vi "load images.vi"(0 "selected data path":path, 1 "DataMarijnFormat":bool=TRUE, 7 "Data(T)orLUT(F)?":bool, 11 "error in":errorcluster, 12 "frame no.":i32) -> (3 "image name":string, 4 "String":string, 6 "Image Out":T1, 10 "framenumber":i32, 14 "error out":errorcluster, 15 "frametime":i32)   [LabVIEW 2011, in "OfflineTracker.lvlib"]
uses:
  <vilib>/vision/Image Controls.llb/IMAQ Image.ctl
  <vilib>/Utility/file.llb/Read From Spreadsheet File (string).vi
  <vilib>/Utility/file.llb/Read From Spreadsheet File (DBL).vi
  OfflineTracker.lvlib
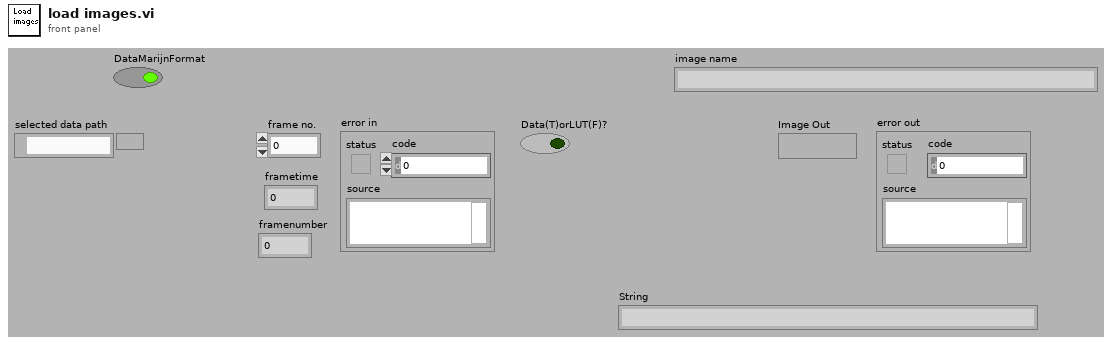
[diagram p1: front panel]
types:
  T1 = typedef "IMAQ Image.ctl" = refnum<image>
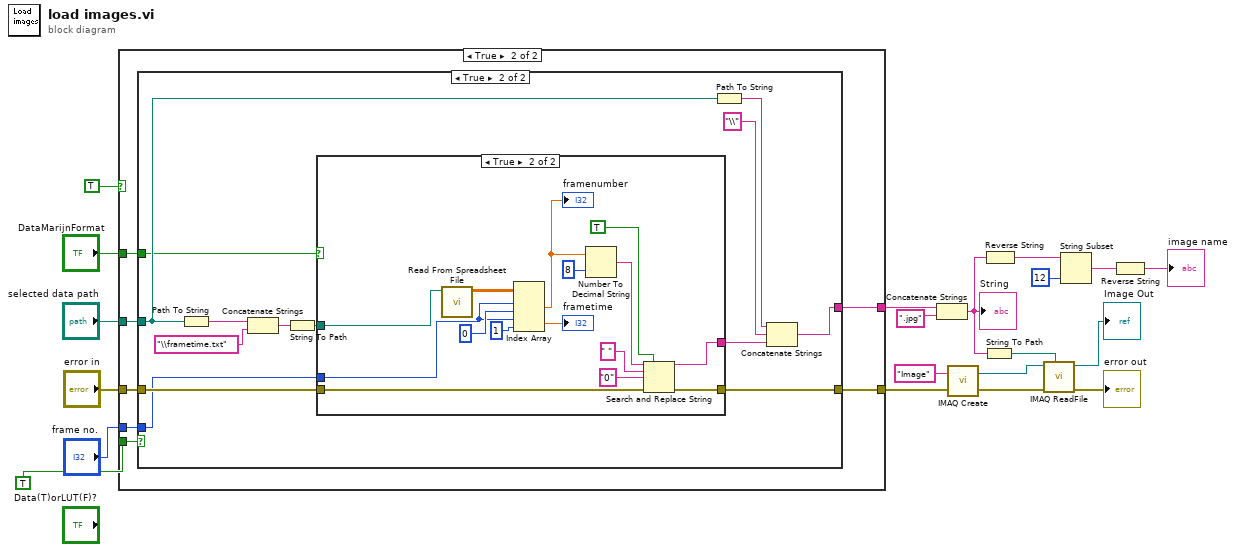
[diagram p0: block diagram]
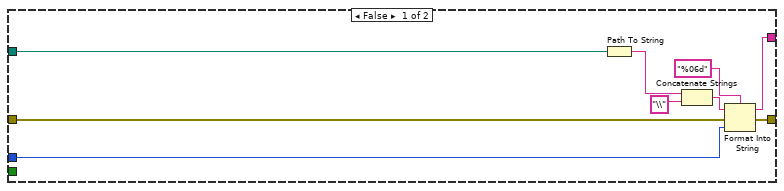
[diagram p2: hidden frame]
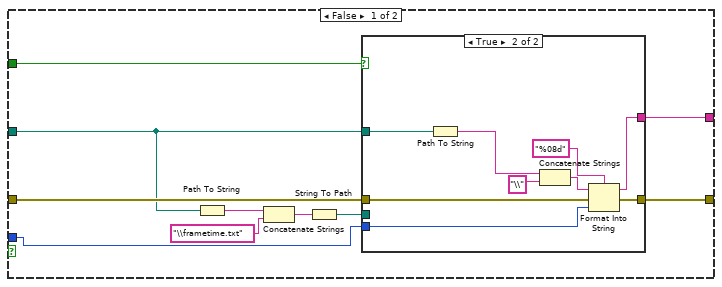
[diagram p3: hidden frame]
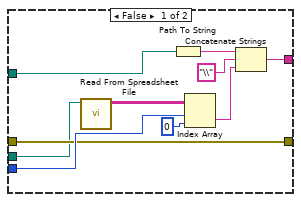
[diagram p4: hidden frame]
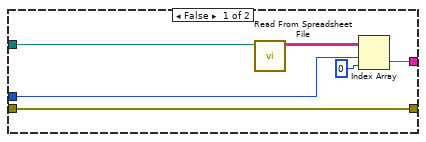
[diagram p5: hidden frame]
diagram:
  n1 = case shown="True" TRUE {
    tunnel: "selected data path" -> [w27 w36]
    tunnel: "error in" -> [w29 w34]
    tunnel: [w28 w33] -> w17
    tunnel: [w26 w35] -> w16
    tunnel: "frame no." -> [w25 w32]
    tunnel: TRUE ("Data(T)orLUT(F)?") -> [_ w31]
    tunnel: "DataMarijnFormat" -> [_ w30]
    frame False {
      n2 = Path To String(path=w27) -> (string=w21:string)
      n3 = Concatenate Strings(w21, "\\" ("string")) -> (w22:string)
      n4 = Format Into String(format string="%06d", initial string=w22, error in=w29, w25) -> (resulting string=w26:string, error out=w28:errorcluster)
    }
    frame True {
      n5 = case shown="True" w31 {
        tunnel: w36 -> [w38 w68]
        tunnel: [w43 w77] -> w35
        tunnel: w34 -> [w46 w74]
        tunnel: [w45 w73] -> w33
        tunnel: w32 -> [w44 w67]
        tunnel: w30 -> [w42 w66]
        frame False {
          n6 = Path To String(path=w38) -> (string=w41:string)
          n7 = Concatenate Strings(w41, "\\frametime.txt" ("string")) -> (w40:string)
          n8 = String To Path(string=w40) -> (path=w37:path)
          n9 = case shown="True" w42 {
            tunnel: w46 -> [w53 w61]
            tunnel: [w53 w60] -> w45
            tunnel: w38 -> [w47 w59]
            tunnel: w44 -> [w54 w58]
            tunnel: [w48 w57] -> w43
            tunnel: w37 -> [w49 _]
            frame False {
              n10 = call-poly <vilib>:"Read From Spreadsheet File.vi"("file path (dialog if empty)"=w49) -> ("all rows"=w56:string[][])  [unwired: 3 in, 7 out]
              n11 = Path To String(path=w47) -> (string=w52:string)
              n12 = Index Array(array=w56, index (row)=w54, index (col)=0 ("disabled index (col)")) -> (element=w50:string)
              n13 = Concatenate Strings(w52, "\\" ("string"), w50) -> (w48:string)
            }
            frame True {
              n14 = Path To String(path=w59) -> (string=w62:string)
              n15 = Concatenate Strings(w62, "\\" ("string")) -> (w63:string)
              n16 = Format Into String(format string="%08d", initial string=w63, error in=w61, w58) -> (resulting string=w57:string, error out=w60:errorcluster)
            }
          }
        }
        frame True {
          n17 = Path To String(path=w68) -> (string=w72:string)
          n18 = Concatenate Strings(w72, "\\frametime.txt" ("string")) -> (w70:string)
          n19 = String To Path(string=w70) -> (path=w71:path)
          n20 = case shown="True" w66 {
            tunnel: [w80 w98] -> w75
            tunnel: w74 -> [w79 w97]
            tunnel: [w79 w96] -> w73
            tunnel: w71 -> [w84 w92]
            tunnel: w67 -> [w81 w90]
            frame False {
              n21 = call-poly <vilib>:"Read From Spreadsheet File.vi"("file path (dialog if empty)"=w84) -> ("all rows"=w83:string[][])  [unwired: 3 in, 7 out]
              n22 = Index Array(array=w83, index (row)=w81, index (col)=0 ("disabled index (col)")) -> (element=w80:string)
            }
            frame True {
              n23 = call-poly <vilib>:"Read From Spreadsheet File.vi"("file path (dialog if empty)"=w92) -> ("all rows"=w91:dbl[][])  [unwired: 3 in, 7 out]
              n24 = Index Array(array=w91, index (row) #1=w90, index (col) #1=0 ("index"), index (row) #2=w90, index (col) #2=1 ("disabled index (col)")) -> (element #1=w99:dbl, element #2=→"frametime":dbl)
              "framenumber" <- w99
              n25 = Number To Decimal String(number=w99, width (-)=i16 8) -> (decimal integer string=w88:string)
              n26 = Search and Replace String(replace all?=TRUE ("replace all? (F)"), input string=w88, search string=" ", replace string="0" ("replace string (\"\")"), error in=w97) -> (result string=w98:string, error out=w96:errorcluster)  [unwired: 5 out]
            }
          }
          n27 = Path To String(path=w68) -> (string=w78:string)
          n28 = Concatenate Strings(w78, "\\" ("string"), w75) -> (w77:string)
        }
      }
    }
  }
  n29 = Concatenate Strings(w16, ".jpg" ("string")) -> (w9:string)
  "String" <- w9
  n30 = call "IMAQ Create"("Image Name"="Image", "error in (no error)"=w17) -> ("New Image"=w11:T1, "error out"=w12:errorcluster)  [unwired: 2 in, 1 out]
  n31 = String To Path(string=w9) -> (path=w15:path)
  n32 = Reverse String(1:w9) -> (0:w8:string)
  n33 = call "IMAQ ReadFile"("File Path"=w15, "error in (no error)"=w12, "Image"=w11) -> ("error out"=→"error out":errorcluster, "Image Out"=→"Image Out":T1)  [unwired: 2 in, 5 out]
  n34 = String Subset(string=w8, length (rest)=12 ("length (rest)")) -> (substring=w6:string)  [unwired: 1 out]
  n35 = Reverse String(1:w6) -> (0:→"image name":string)
